vi "Set Time Scale.vi"(8 "TRIARC_ERROR_IN":errorcluster, 10 "Time Scale [ms]":u32, 11 "Person In":refnum<class "Person.lvclass">) -> (0 "TRIARC_ERROR_OUT":errorcluster, 3 "Person Out":refnum<class "Person.lvclass">)   [LabVIEW 2020, in "Person.lvclass"]
uses:
  Person.lvclass
  C:/Program Files (x86)/National Instruments/LabVIEW 2020/vi.lib/Astemes/Triarc Framework/Process/Process.lvclass
  <vilib>/Astemes/Triarc Framework/Process/Process.lvclass/Process.ctl
  Person.lvclass/Person.ctl
  <vilib>/Astemes/Triarc Framework/Process/Private/SubVIs/Handle Debug Data.vi
  <vilib>/Astemes/Triarc Framework/Logging/Log Debug.vi
  <vilib>/AdvancedString/1D String Array to Delimited String.vi
  <vilib>/Utility/High Resolution Relative Seconds.vi
  <vilib>/Astemes/Triarc Framework/Process/Public/Read Name.vi
  <vilib>/Astemes/Triarc Framework/Callback/Callback.lvclass
  <vilib>/Astemes/Triarc Framework/Process/Process.lvclass
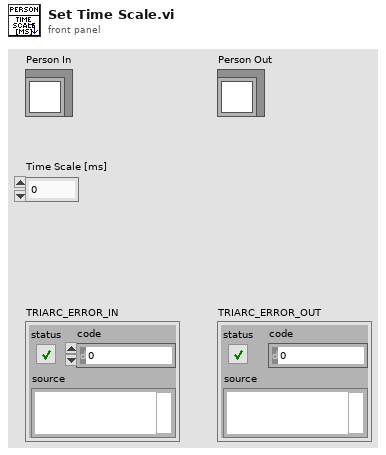
[diagram p1: front panel]
types:
  T1 = typedef "TF.lvlib/Process.lvclass/API Mode.ctl" = enum16{"Send Message", "Handle Message"}
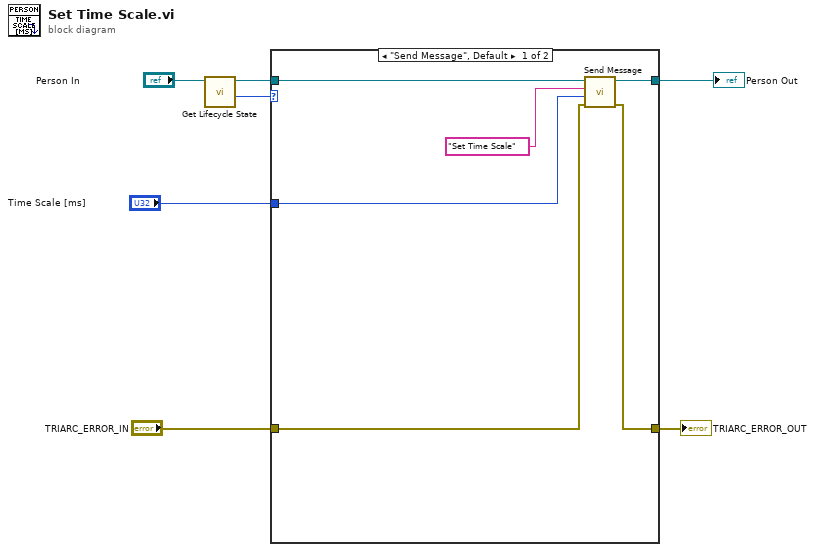
[diagram p0: block diagram]
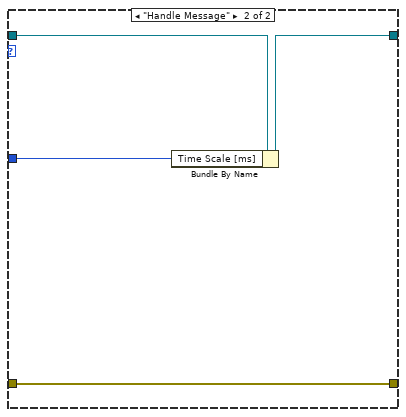
[diagram p2: hidden frame]
diagram:
  n1 = call <vilib>:"Get Lifecycle State.vi"("Process In"="Person In") -> ("API Mode"=w3:T1, "Process Out"=w6:refnum<class "Person.lvclass">)  [unwired: 7 in, 2 out]
  n2 = case shown="\"Send Message\", Default" w3 {
    tunnel: w6 -> [w13 w17]
    tunnel: [w12 w15] -> w5
    tunnel: "TRIARC_ERROR_IN" -> [w8 w16]
    tunnel: [w9 w16] -> w4
    tunnel: "Time Scale [ms]" -> [w11 w14]
    frame "Send Message", Default {
      n3 = call <vilib>:"Send Message.vi"("error in (no error)"=w8, "Message Data"=w11, "Message"="Set Time Scale" ("API Message"), "Process In"=w13) -> ("error out"=w9:errorcluster, "Process Out"=w12:refnum<class "Person.lvclass">)  [unwired: 6 in]
    }
    frame "Handle Message" {
      n4 = Bundle By Name(cluster=w17, "Time Scale [ms]"=w14) -> (w15:refnum<class "Person.lvclass">)
    }
  }
  "TRIARC_ERROR_OUT" <- w4
  "Person Out" <- w5
